vi "GVmotor_auto_ctrl_with_pressure.vi"(6 "ref_turn_set":refnum<vi>, 7 "array_value_in":dbl[](array[numeric]), 9 "P_set":dbl=10.0 caption="Set Point" format="%#_13g", 10 "enable_auto_ctrl":bool caption="Auto Control\nwith Pressure") -> (0 "turn_new":dbl format="%.3f", 1 "auto_ctrl_status":u32(colorbox) caption="Status", 3 "P_now":dbl format="%.2f", 5 "array_value_out":dbl[](array[numeric]))   [LabVIEW 2019]
doc: "This example demonstrates how to simulate a general PID controller."
uses:
  <vilib>/Analysis/baseanly.llb/Mean (DBL).vi
  MKS670/MKS670_Global.vi
  <vilib>/addons/control/pid/pid.llb/PID (DBL).vi
  <vilib>/addons/control/pid/NI_PID_pid.lvlib
  <vilib>/Analysis/NI_AALBase.lvlib
panel:
  in  "sp_step":dbl=0.001 format="%#_13g"
  in  "sp_nominal":dbl=0.03
  in  "sp_max":dbl=0.25
  in  "sp_min":dbl
  in  "n_avg":u8=4
  out "MV":dbl format="%.1f"
  in  "P_max":dbl=500.0 format="%.1f"
  in  "P_min":dbl=-10.0 format="%.1f"
  out "PID Range":cluster{"High":dbl, "Low":dbl} {"Low" format="%.1f"; "High" format="%.1f"}
  in  "PID gains":T1={"proportional gain (Kc)"=-0.001, "integral time (Ti, min)"=0.3, "derivative time (Td, min)"=0.1} {"derivative time (Td, min)" format="%.4f"; "integral time (Ti, min)" format="%.4f"; "proportional gain (Kc)" format="%.3f"}
  # "Torr"
  # "Torr"
  # "Torr"
  # "K_c = dT/dP = -0.001/1 = -0.001\nT_i = 0.5\nT_d = 0.1"
  # "The parameters were last modified on 2024-01-06."
  # "L/m"
  # "L/m"
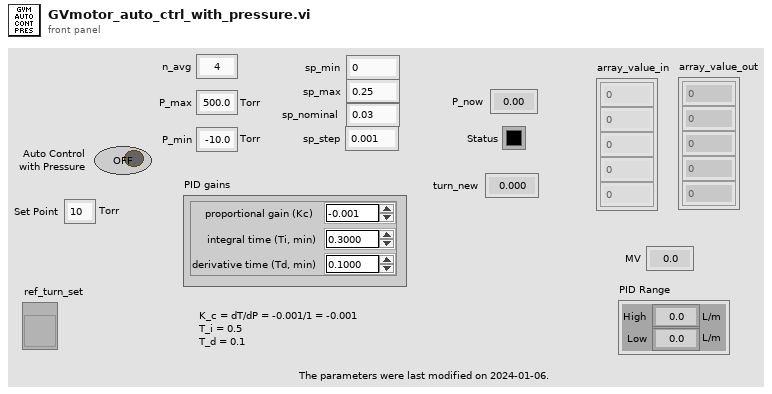
[diagram p1: front panel]
types:
  T1 = cluster{"proportional gain (Kc)":dbl, "integral time (Ti, min)":dbl, "derivative time (Td, min)":dbl}
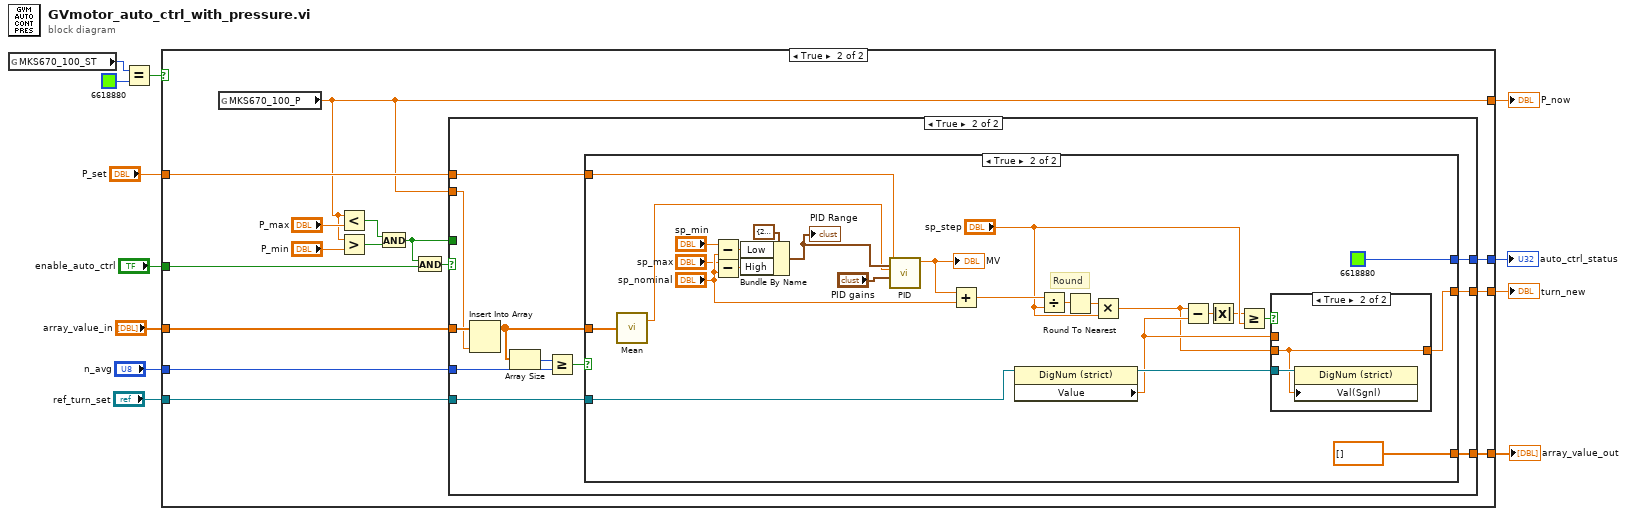
[diagram p0: block diagram]
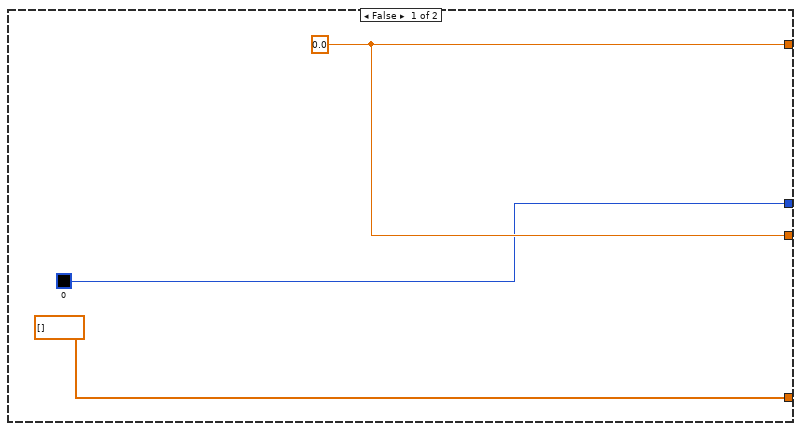
[diagram p2: hidden frame]
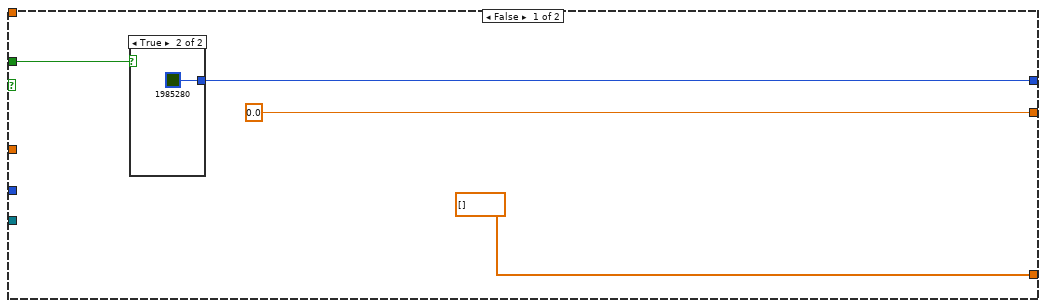
[diagram p3: hidden frame]
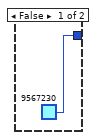
[diagram p4: hidden frame]
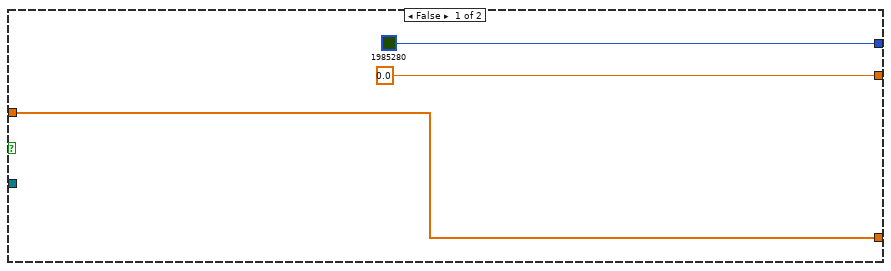
[diagram p5: hidden frame]
diagram:
  n1 = global read "MKS670_Global.vi" "MKS670_100_ST"() -> (w1:u32)
  n2 = Equal?(x=w1, y=u32 6618880 ("MG_ST")) -> (x = y?=w2:bool)
  n3 = case shown="True" w2 {
    tunnel: [w15 w30] -> w12
    tunnel: [u32 0 ("alarm_status") w29] -> w11
    tunnel: "P_set" -> [_ w20]
    tunnel: "enable_auto_ctrl" -> [_ w24]
    tunnel: [w15 w16] -> w8
    tunnel: "ref_turn_set" -> [_ w26]
    tunnel: "array_value_in" -> [_ w19]
    tunnel: "n_avg" -> [_ w18]
    tunnel: [dbl[] [] ("f") w17] -> w4
    frame False {
      w15 = 0.0 ("Value")
    }
    frame True {
      n4 = global read "MKS670_Global.vi" "MKS670_100_P"() -> (w16:dbl)
      n5 = Less?(x=w16, y="P_max") -> (x < y?=w22:bool)
      n6 = Greater?(x=w16, y="P_min") -> (0:w23:bool)
      n7 = And(x=w22, y=w23) -> (x .and. y?=w21:bool)
      n8 = And(x=w21, y=w24) -> (x .and. y?=w25:bool)
      n9 = case shown="True" w25 {
        tunnel: [0.0 ("F_O_new") w45] -> w30
        tunnel: [w32 w47] -> w29
        tunnel: w20 -> [_ w44]
        tunnel: w16 -> [_ w42]
        tunnel: w26 -> [_ w46]
        tunnel: w21 -> [w33 _]
        tunnel: w19 -> [_ w43]
        tunnel: w18 -> [_ w40]
        tunnel: [dbl[] [] ("f") w37] -> w17
        frame False {
          n10 = case shown="True" w33 {
            tunnel: [u32 9567230 ("alarm_status") u32 1985280 ("alarm_status")] -> w32
            frame False {
            }
            frame True {
            }
          }
        }
        frame True {
          n11 = Insert Into Array(array=w43, new element=w42) -> (w38:dbl[])  [unwired: 1 in]
          n12 = Array Size(array=w38) -> (size(s)=w41:i32)
          n13 = Greater Or Equal?(x=w41, y=w40) -> (x >= y?=w39:bool)
          n14 = case shown="True" w39 {
            tunnel: [u32 1985280 ("alarm_status") u32 6618880 ("alarm_status")] -> w47
            tunnel: w46 -> [_ w75]
            tunnel: [0.0 ("F_new") w74] -> w45
            tunnel: w44 -> [_ w72]
            tunnel: w38 -> [w48 w63]
            tunnel: [w48 dbl[] [] ("f")] -> w37
            frame False {
            }
            frame True {
              # "Round"
              n15 = call-poly <vilib>:"Mean.vi"("X"=w63) -> ("mean"=w62:dbl)  [unwired: 1 out]
              n16 = Subtract(x="sp_min", y="sp_nominal") -> (x-y=w68:dbl)
              n17 = Subtract(x="sp_max", y="sp_nominal") -> (x-y=w69:dbl)
              n18 = Bundle By Name(cluster=cluster{"High":dbl, "Low":dbl} {"High"=20.0, "Low"=-20.0} ("PID Range"), "Low"=w68, "High"=w69) -> (w64:cluster{"High":dbl, "Low":dbl})
              "PID Range" <- w64
              n19 = call-poly <vilib>:"PID.vi"("output range"=w64, "PID gains"="PID gains", "process variable"=w62, "setpoint"=w72) -> ("output"=w71:dbl)  [unwired: 6 in, 1 out]
              "MV" <- w71
              n20 = Add(x=w71, y="sp_nominal") -> (x+y=w58:dbl)
              n21 = property class="DigNum (strict)"(reference=w75) -> ("Value"=w60:dbl)  [unwired: 1 in, 2 out]
              n22 = Divide(x=w58, y="sp_step") -> (x/y=w55:dbl)
              n23 = Round To Nearest(number=w55) -> (nearest integer value=w56:dbl)
              n24 = Multiply(x=w56, y="sp_step") -> (x*y=w59:dbl)
              n25 = Subtract(x=w59, y=w60) -> (x-y=w52:dbl)
              n26 = Absolute Value(x=w52) -> (abs(x)=w53:dbl)
              n27 = Greater Or Equal?(x=w53, y="sp_step") -> (x >= y?=w54:bool)
              n28 = case shown="True" w54 {
                tunnel: w75 -> [_ w78]
                tunnel: w59 -> [_ w77]
                tunnel: [w76 w77] -> w74
                tunnel: w60 -> [w76 _]
                frame False {
                }
                frame True {
                  n29 = property class="DigNum (strict)"(reference=w78, "Val(Sgnl)"=w77) -> ()  [unwired: 1 in, 2 out]
                }
              }
            }
          }
        }
      }
    }
  }
  "turn_new" <- w12
  "auto_ctrl_status" <- w11
  "P_now" <- w8
  "array_value_out" <- w4
